vi "Read.vi"(8 "error in (no error)":errorcluster, 11 "Parallax PING))) in":refnum<class "Parallax PING))).lvclass">) -> (0 "error out":errorcluster, 1 "Timed out?":bool, 2 "Distance (m)":dbl, 3 "Parallax PING))) out":refnum<class "Parallax PING))).lvclass">)   [LabVIEW 2013, in "Parallax PING))).lvclass"]
doc: "Reads the distance in m."
uses:
  Parallax PING))).lvclass
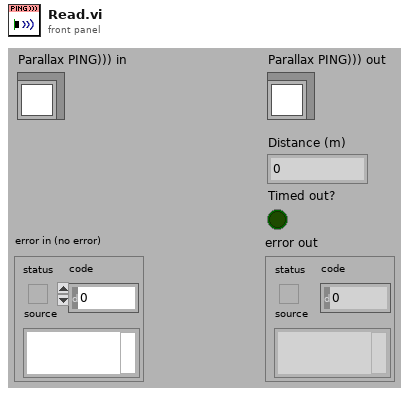
[diagram p1: front panel]
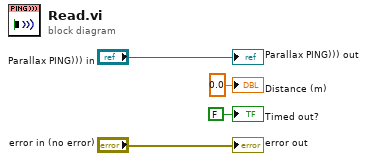
[diagram p0: block diagram]
diagram:
  "error out" <- "error in (no error)"
  "Parallax PING))) out" <- "Parallax PING))) in"
  "Distance (m)" <- 0.0 ("Distance (m)")
  "Timed out?" <- FALSE ("Timed out?")
